vi "spectrum_analyzer_labview.vi"() -> ()   [LabVIEW 2023]
uses:
  <vilib>/sound2/lvsound2.llb/Sound Data Format.ctl
  <vilib>/sound2/lvsound2.llb/Sound File Write Open.vi
  <vilib>/express/express analysis/Spectral/Block/exnSpectralBlock spectral measurements RMS poly.vi
  <vilib>/express/express analysis/Spectral/Block/exnSpectralBlock spectral measurements RMS DDT.vi
  <vilib>/sound2/lvsound2.llb/Sound File Write (DBL).vi
  <vilib>/express/express analysis/Spectral/XNode/ExpressSpectralMeasurementsBlockNode.xnode
panel:
  out "Generated Sound File":path
  out "Sharp Indicator":string="\n\n            SHARP"
  out "Flat Indicator":string="\n\n             FLAT"
  out "Note Played":string
  in  "Notes":string[](array[string])=["C0", "C#/Db0", "D0", "D#/Eb0", "E0", "F0", "F#/Gb0", "G0", "G#/Ab0", "A0", "A#/Bb0", "B0", "C1", "C#/Db1", "D1", "D#/Eb1", "E1", "F1", "F#/Gb1", "G1", "G#/Ab1", "A1", "A#/Bb1", "B1", "C2", "C#/Db2", "D2", "D#/Eb2", "E2", "F2", "F#/Gb2", "G2", "G#/Ab2", "A2", "A#/Bb2", "B2", "C3", "C#/Db3", "D3", "D#/Eb3", "E3", "F3", "F#/Gb3", "G3", "G#/Ab3", "A3", "A#/Bb3", "B3", "C4", "C#/Db4", "D4", "D#/Eb4", "E4", "F4", "F#/Gb4", "G4", "G#/Ab4", "A4", "A#/Bb4", "B4", "C5", "C#/Db5", "D5", "D#/Eb5", "E5", "F5", "F#/Gb5", "G5", "G#/Ab5", "A5", "A#/Bb5", "B5", "C6", "C#/Db6", "D6", "D#/Eb6", "E6", "F6", "F#/Gb6", "G6", "G#/Ab6", "A6", "A#/Bb6", "B6", "C7", "C#/Db7", "D7", "D#/Eb7", "E7", "F7", "F#/Gb7", "G7", "G#/Ab7", "A7", "A#/Bb7", "B7", "C8", "C#/Db8", "D8", "D#/Eb8", "E8", "F8", "F#/Gb8", "G8", "G#/Ab8", "A8", "A#/Bb8", "B8"]
  in  "Note Frequencies":dbl[](array[numeric])=[16.35, 17.32, 18.35, 19.45, 20.6, 21.83, 23.12, 24.5, 25.96, 27.5, 29.14, 30.87, 32.7, 34.65, 36.71, 38.89, 41.2, 43.65, 46.25, 49.0, 51.91, 55.0, 58.27, 61.74, 65.41, 69.3, 73.42, 77.78, 82.41, 87.31, 92.5, 98.0, 103.83, 110.0, 116.54, 123.47, 130.81, 138.59, 146.83, 155.56, 164.81, 174.61, 185.0, 196.0, 207.65, 220.0, 233.08, 246.94, 261.63, 277.18, 293.66, 311.13, 329.63, 349.23, 369.99, 392.0, 415.3, 440.0, 466.16, 493.88, 523.25, 554.37, 587.33, 622.25, 659.25, 698.46, 739.99, 783.99, 830.61, 880.0, 932.33, 987.77, 1046.5, 1108.73, 1174.66, 1244.51, 1318.51, 1396.91, 1479.98, 1567.98, 1661.22, 1760.0, 1864.66, 1975.53, 2093.0, 2217.46, 2349.32, 2489.02, 2637.02, 2793.83, 2959.96, 3135.96, 3322.44, 3520.0, 3729.31, 3951.07, 4186.01, 4434.92, 4698.63, 4978.03, 5274.04, 5587.65, 5919.91, 6271.93, 6644.88, 7040.0, 7458.62, 7902.13]
  out "Frequency, Hz":i32
  in  "Start/Stop Recording":bool
  in  "Test Loudness":dbl(slide) scale=0.0..140.0
  in  "Simulate Loudness":bool
  out "Safe for:":string
  out "OSHA Equiv. Sound Level":string
  out "dB SPL":dbl
  out "dB SPL Meter":dbl(knob)=60.264729150013714 scale=0.0..140.0
  in  "Quit App":bool
  out "Fast Fourier Transform":dynamicdata(graph)
  out "Raw Sound":dynamicdata(graph) caption="Data"
  # "LOUDNESS METER"
  # "ELECTRIC TUNER"
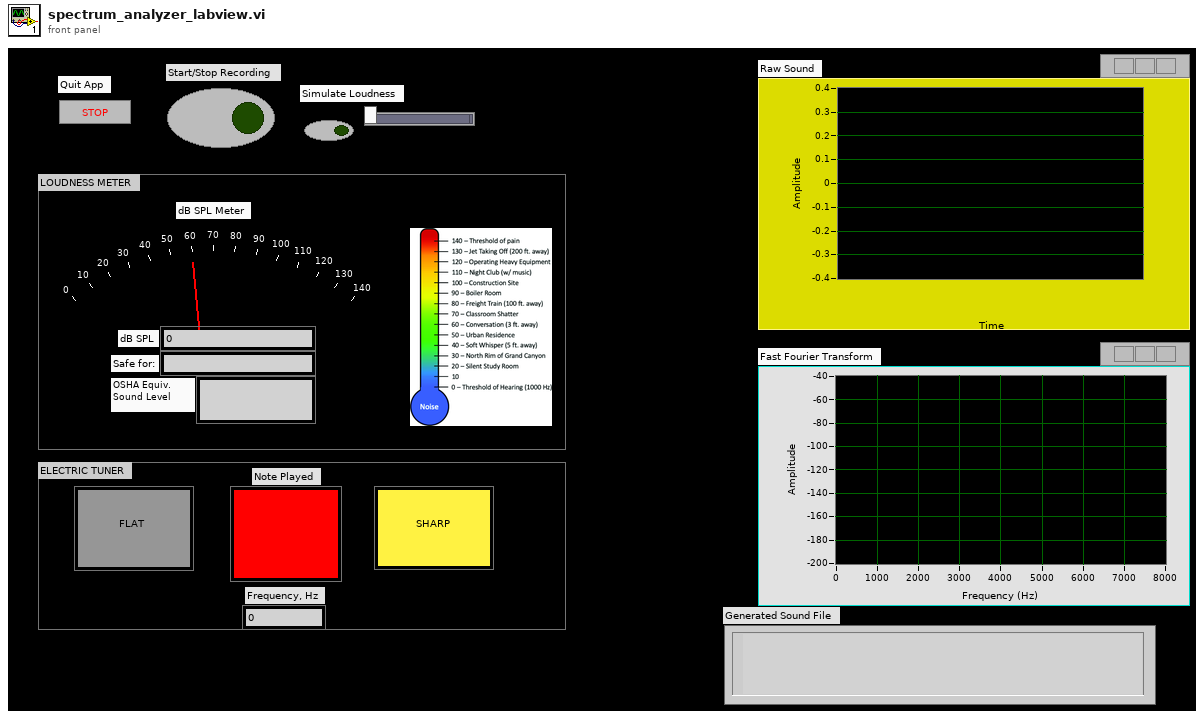
[diagram p1: front panel]
types:
  T1 = typedef "Sound Data Format.ctl" = cluster{"sample rate (S/s)":dbl, "number of channels":i32, "bits per sample":i32}
  T2 = typedef "Sound File Refnum.ctl" = refnum<file>
  T3 = cluster{"averaging mode":u16, "weighting mode":u16, "number of averages":u32}
  T4 = cluster{"dB On (F)":bool, "unwrap phase (F)":bool, "convert to degree (F)":bool}
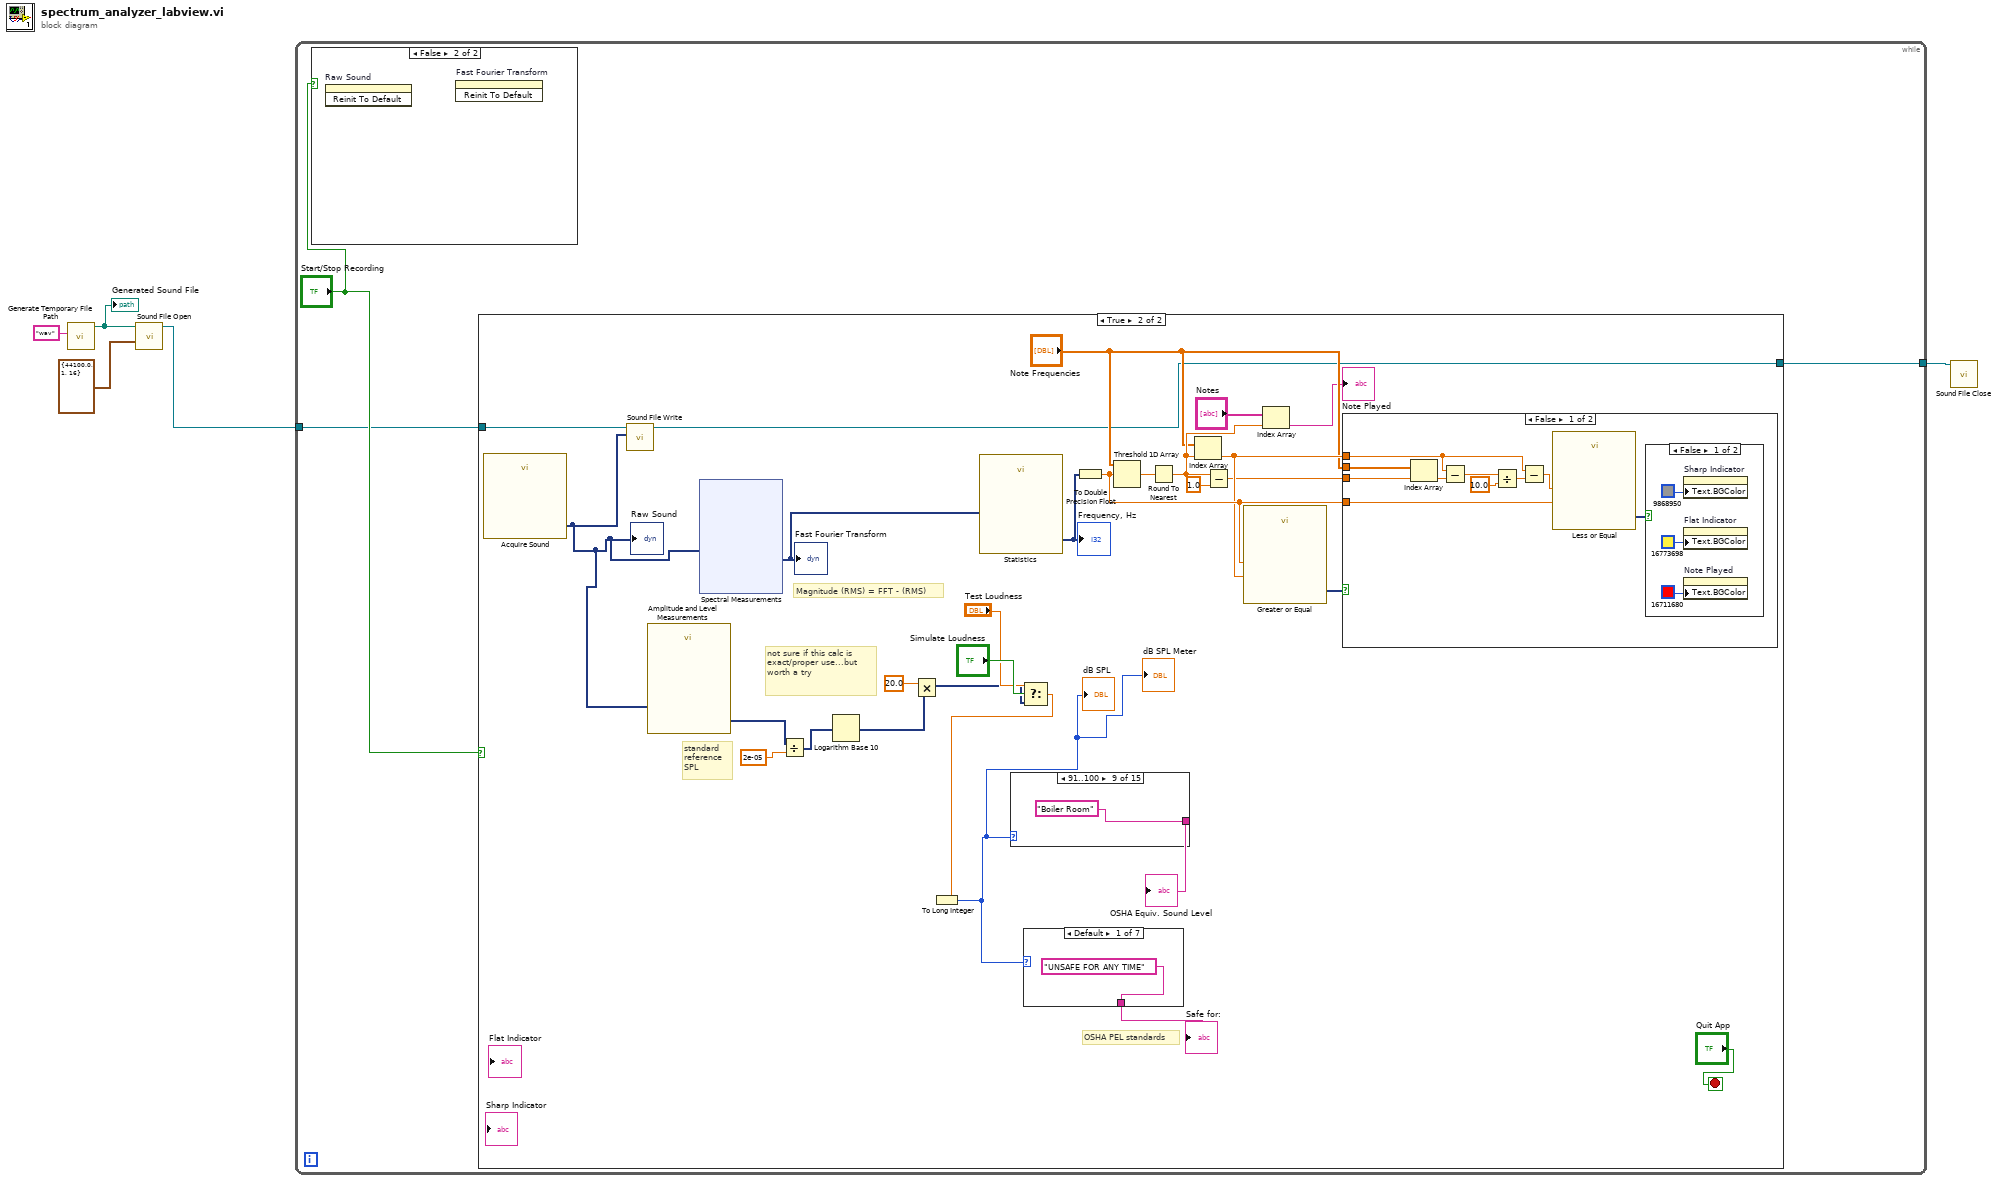
[diagram p0: block diagram]
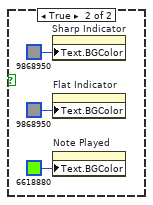
[diagram p4: hidden frame]
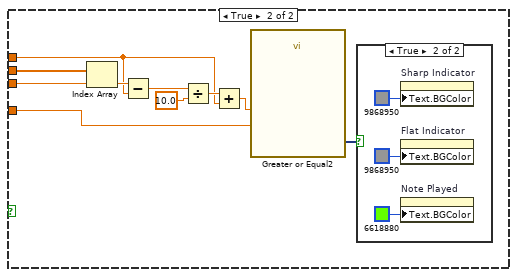
[diagram p5: hidden frame]
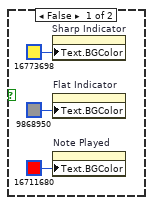
[diagram p6: hidden frame]
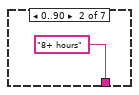
[diagram p7: hidden frame]
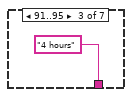
[diagram p8: hidden frame]
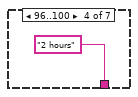
[diagram p9: hidden frame]
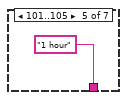
[diagram p10: hidden frame]
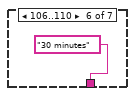
[diagram p11: hidden frame]
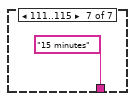
[diagram p12: hidden frame]
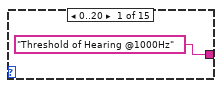
[diagram p13: hidden frame]
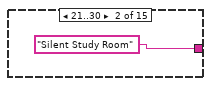
[diagram p14: hidden frame]
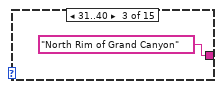
[diagram p15: hidden frame]
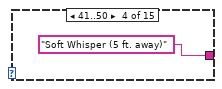
[diagram p16: hidden frame]
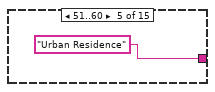
[diagram p17: hidden frame]
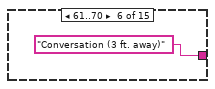
[diagram p18: hidden frame]
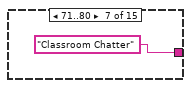
[diagram p19: hidden frame]
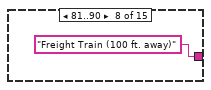
[diagram p20: hidden frame]
diagram:
  n1 = call <vilib>:"Generate Temporary File Path.vi"("Temporary File Extension (tmp)"="wav") -> ("Unique Temporary File Path"=w5:path)  [unwired: 9 in, 1 out]
  "Generated Sound File" <- w5
  n2 = call-poly <vilib>:"Sound File Open.vi"("sound format"=T1 {"sample rate (S/s)"=44100.0, "number of channels"=1, "bits per sample"=16} ("Sound Format"), "path"=w5) -> ("sound file refnum"=w2:T2)  [unwired: 8 in, 1 out]
  n3 = while {
    tunnel: w2 -> [w7]
    tunnel: [w6] -> w1
    stop <- "Quit App" stop-if-true
    n4 = case shown="False" "Start/Stop Recording" {
      frame True {
      }
      frame False {
        n5 = invoke on="Raw Sound" class="WFGraph (strict)" method="Reinit To Default"() -> ()  [unwired: 3 in, 3 out]
        n6 = invoke on="Fast Fourier Transform" class="WFGraph (strict)" method="Reinit To Default"() -> ()  [unwired: 3 in, 3 out]
      }
    }
    n7 = case shown="True" "Start/Stop Recording" {
      tunnel: w7 -> [w10 w12]
      tunnel: [w10 w11] -> w6
      frame False {
      }
      frame True {
        # "OSHA PEL standards"
        # "standard reference SPL"
        # "not sure if this calc is exact/proper use...but worth a try"
        # "Magnitude (RMS) = FFT - (RMS)"
        n8 = call "Acquire Sound"() -> ("Data"=w13:dynamicdata)  [unwired: 18 in, 1 out]
        "Raw Sound" <- w13
        n9 = call-poly <vilib>:"Sound File Write.vi"("data"=w13, "sound file refnum"=w12) -> ("sound file refnum out"=w11:T2)  [unwired: 8 in, 1 out]
        n10 = call "Amplitude and Level Measurements"("Signals"=w13) -> ("RMS"=w34:dynamicdata)  [unwired: 13 in, 1 out]
        n11 = xnode "Spectral Measurements"("Signals"=w13) -> ("FFT - (RMS)"=w14:dynamicdata)  [unwired: 1 in, 2 out]
        "Fast Fourier Transform" <- w14
        n12 = Divide(x=w34, y=2e-05) -> (x/y=w35:dynamicdata)
        n13 = Logarithm Base 10(1:w35) -> (0:w36:dynamicdata)
        n14 = Multiply(x=20.0, y=w36) -> (x*y=w28:dynamicdata)
        n15 = call "Statistics"("Signals"=w14) -> ("Time of Maximum"=w16:dynamicdata)  [unwired: 24 in, 2 out]
        "Frequency, Hz" <- w16
        n16 = Select(t="Test Loudness", s="Simulate Loudness", f=w28) -> (s? t:f=w27:dbl)
        n17 = To Long Integer(number=w27) -> (32bit integer=w26:i32)
        "dB SPL Meter" <- w26
        "dB SPL" <- w26
        n18 = case shown="91..100" w26 {
          tunnel: ["Threshold of Hearing @1000Hz" "Silent Study Room" "North Rim of Grand Canyon" "Soft Whisper (5 ft. away)" "Urban Residence" "Conversation (3 ft. away)" "Classroom Chatter" "Freight Train (100 ft. away)" "Boiler Room" "Construction Site" "Night Club (w/ music)" "Unsafe!" "Operating Heavy Equipment" "Jet Taking Off (200 ft. away)" "Threshold of pain"] -> w32
          frame 0..20 {
          }
          frame 21..30 {
          }
          frame 31..40 {
          }
          frame 41..50 {
          }
          frame 51..60 {
          }
          frame 61..70 {
          }
          frame 71..80 {
          }
          frame 81..90 {
          }
          frame 91..100 {
          }
          frame 101..110 {
          }
          frame 111..120 {
          }
          frame Default {
          }
          frame 121..130 {
          }
          frame 131..140 {
          }
          frame 141.. {
          }
        }
        "OSHA Equiv. Sound Level" <- w32
        n19 = case shown="Default" w26 {
          tunnel: ["UNSAFE FOR ANY TIME" "8+ hours" "4 hours" "2 hours" "1 hour" "30 minutes" "15 minutes"] -> w31
          frame Default {
          }
          frame 0..90 {
          }
          frame 91..95 {
          }
          frame 96..100 {
          }
          frame 101..105 {
          }
          frame 106..110 {
          }
          frame 111..115 {
          }
        }
        "Safe for:" <- w31
        n20 = To Double Precision Float(number=w16) -> (double precision float=w24:dbl)
        n21 = Threshold 1D Array(2:w24, 3:"Note Frequencies") -> (0:w17:dbl)  [unwired: 1 in]
        n22 = Round To Nearest(number=w17) -> (nearest integer value=w25:dbl)
        n23 = Index Array(array="Note Frequencies", index=w25) -> (element=w23:dbl)
        n24 = Subtract(x=w25, y=1.0 ("x")) -> (x-y=w21:dbl)
        n25 = call "Greater or Equal"("Operand 2"=w23, "Operand 1"=w24) -> ("Result"=w19:dynamicdata)  [unwired: 8 in, 1 out]
        n26 = Index Array(array="Notes", index=w25) -> (element=→"Note Played":string)
        n27 = case shown="False" w19 {
          tunnel: w21 -> [w43 w63]
          tunnel: "Note Frequencies" -> [w42 w62]
          tunnel: w23 -> [w39 w56]
          tunnel: w24 -> [w38 w54]
          frame False {
            n28 = Index Array(array=w42, index=w43) -> (element=w41:dbl)
            n29 = Subtract(x=w39, y=w41) -> (x-y=w45:dbl)
            n30 = Divide(x=w45, y=10.0) -> (x/y=w40:dbl)
            n31 = Subtract(x=w39, y=w40) -> (x-y=w46:dbl)
            n32 = call "Less or Equal"("Operand 2"=w38, "Operand 1"=w46) -> ("Result"=w47:dynamicdata)  [unwired: 8 in, 1 out]
            n33 = case shown="False" w47 {
              frame False {
                n34 = property on="Sharp Indicator" class="Str"("Text.BGColor"=u32 9868950) -> ()  [unwired: 2 in, 2 out]
                n35 = property on="Flat Indicator" class="Str"("Text.BGColor"=u32 16773698) -> ()  [unwired: 2 in, 2 out]
                n36 = property on="Note Played" class="Str"("Text.BGColor"=u32 16711680) -> ()  [unwired: 2 in, 2 out]
              }
              frame True {
                n37 = property on="Sharp Indicator" class="Str"("Text.BGColor"=u32 9868950) -> ()  [unwired: 2 in, 2 out]
                n38 = property on="Flat Indicator" class="Str"("Text.BGColor"=u32 9868950) -> ()  [unwired: 2 in, 2 out]
                n39 = property on="Note Played" class="Str"("Text.BGColor"=u32 6618880) -> ()  [unwired: 2 in, 2 out]
              }
            }
          }
          frame True {
            n40 = Index Array(array=w62, index=w63) -> (element=w61:dbl)
            n41 = Subtract(x=w61, y=w56) -> (x-y=w60:dbl)
            n42 = Divide(x=w60, y=10.0) -> (x/y=w58:dbl)
            n43 = Add(x=w58, y=w56) -> (x+y=w57:dbl)
            n44 = call "Greater or Equal2"("Operand 2"=w54, "Operand 1"=w57) -> ("Result"=w55:dynamicdata)  [unwired: 8 in, 1 out]
            n45 = case shown="True" w55 {
              frame False {
                n46 = property on="Sharp Indicator" class="Str"("Text.BGColor"=u32 16773698) -> ()  [unwired: 2 in, 2 out]
                n47 = property on="Flat Indicator" class="Str"("Text.BGColor"=u32 9868950) -> ()  [unwired: 2 in, 2 out]
                n48 = property on="Note Played" class="Str"("Text.BGColor"=u32 16711680) -> ()  [unwired: 2 in, 2 out]
              }
              frame True {
                n49 = property on="Sharp Indicator" class="Str"("Text.BGColor"=u32 9868950) -> ()  [unwired: 2 in, 2 out]
                n50 = property on="Flat Indicator" class="Str"("Text.BGColor"=u32 9868950) -> ()  [unwired: 2 in, 2 out]
                n51 = property on="Note Played" class="Str"("Text.BGColor"=u32 6618880) -> ()  [unwired: 2 in, 2 out]
              }
            }
          }
        }
      }
    }
  }
  n52 = call <vilib>:"Sound File Close.vi"("sound file refnum"=w1) -> ()  [unwired: 10 in, 1 out]
